vi "Configure AM Enabled [AM].vi"(8 "error in (no error)":errorcluster, 9 "AM enabled (True)":bool=TRUE, 10 "Channel Name (\"\")":string="CHANNEL1" caption="channel name (\"CHANNEL1\")", 11 "CS++Fgen in":refnum<class "CS++Fgen.lvclass">) -> (0 "error out":errorcluster, 3 "CS++Fgen out":refnum<class "CS++Fgen.lvclass">)   [LabVIEW 2013, in "CS++Fgen.lvlib" / "CS++Fgen.lvclass"]
doc: "This VI configures whether the function generator applies amplitude modulation to the channel.\n\nNotes:\n\n(1) This VI is part of the IviFgenModulateAM [AM] extension group."
uses:
  CS++Fgen.lvclass
  Core/Classes/CS++ProcessVariables/ProcessVariable/PV.lvclass
  Core/Classes/CS++ProcessVariables/ProcessVariable/PV.lvclass/PV.ctl
  CS++Fgen.lvclass/CS++Fgen.ctl
  Core/Classes/CS++ProcessVariables/PVConnection/PVConnection.lvclass
  Core/Classes/CS++ProcessVariables/ProcessVariable/Write Data.vi
  Core/Classes/CS++ProcessVariables/ProcessVariable/Write Timestamp.vi
  Core/Classes/CS++ProcessVariables/ProcessVariable/Write Quality.vi
  Core/Classes/CS++ProcessVariables/ProcessVariable/Write status.vi
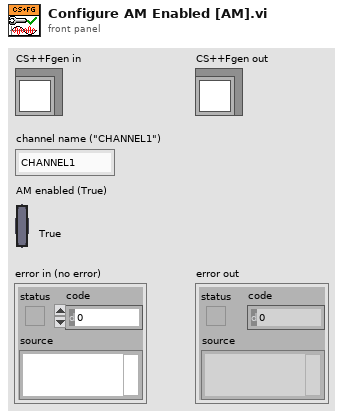
[diagram p1: front panel]
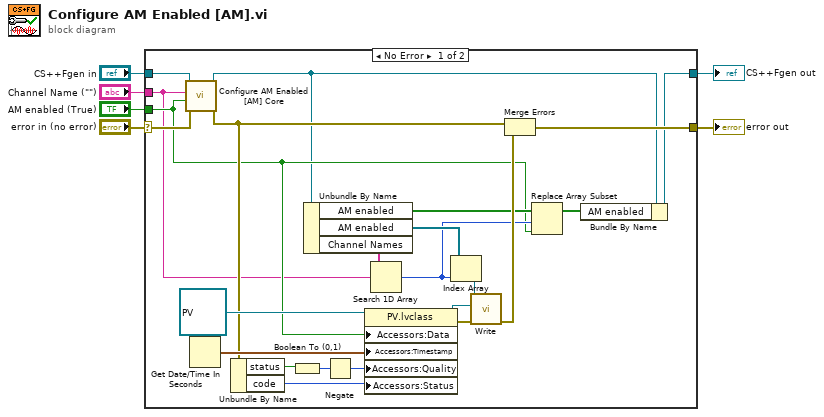
[diagram p0: block diagram]
diagram:
  n1 = case shown="No Error" "error in (no error)" {
    selector: "error in (no error)" -> [w28 w31]
    tunnel: [w11 w31] -> w5
    tunnel: [w7 w30] -> w3
    tunnel: "CS++Fgen in" -> [w29 w30]
    tunnel: "Channel Name (\"\")" -> [w9 _]
    tunnel: "AM enabled (True)" -> [w10 _]
    frame No Error {
      n2 = call-dynamic "Configure AM Enabled [AM] Core.vi"("error in (no error)"=w28, "AM enabled (True)"=w10, "Channel Name (\"\")"=w9, "CS++Fgen in"=w29) -> ("error out"=w12:errorcluster, "CS++Fgen out"=w8:refnum<class "CS++Fgen.lvclass">)  [unwired: 6 in]
      n3 = Get Date/Time In Seconds() -> (seconds since 1Jan1904=w27:timestamp)
      n4 = Unbundle By Name(w12) -> ("status"=w19:bool, "code"=w17:i32)
      n5 = Boolean To (0,1)(Boolean=w19) -> (0, 1=w18:i16)
      n6 = Unbundle By Name(w8) -> ("AM enabled"=w15:bool[], "AM enabled"=w22:refnum<class "PVConnection.lvclass">[], "Channel Names"=w23:string[])
      n7 = Negate(x=w18) -> (-x=w16:i16)
      n8 = property class="PV.lvclass"(reference=refnum<class "PV.lvclass"> refnum ("PV"), "Accessors:Data"=w10, "Accessors:Timestamp"=w27, "Accessors:Quality"=w16, "Accessors:Status"=w17) -> (reference out=w24:refnum<class "PV.lvclass">, error out=w25:errorcluster)  [unwired: 1 in]
      n9 = Search 1D Array(1D array=w23, element=w9) -> (index of element=w13:i32)  [unwired: 1 in]
      n10 = Index Array(array=w22, index=w13) -> (element=w21:refnum<class "PVConnection.lvclass">)
      n11 = call-dynamic "Write.vi"("error in (no error)"=w25, "PV"=w24, "PVConnection in"=w21) -> ("error out"=w20:errorcluster)  [unwired: 7 in, 1 out]
      n12 = Merge Errors(w12, w20) -> (w11:errorcluster)
      n13 = Replace Array Subset(array=w15, new element=w10, index=w13) -> (w14:bool[])
      n14 = Bundle By Name(cluster=w8, "AM enabled"=w14) -> (w7:refnum<class "CS++Fgen.lvclass">)
    }
    frame Error {
    }
  }
  "error out" <- w5
  "CS++Fgen out" <- w3
